vi "startdelayLUT_coMD.vi"() -> ()   [LabVIEW 2012]
doc: "SciScan 1.2 160622"
uses:
  <vilib>/Utility/VariantDataType/Type.ctl
  GFG/GFGbooleanGet.vi
  GFG/GFGfpRefGet.vi
  GFG/GFGstringGet.vi
  GFG/GFG library.lvlib
  <vilib>/Utility/VariantDataType/VariantType.lvlib
panel:
  out "error out 2":errorcluster
  out "error out":errorcluster
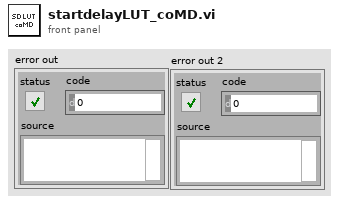
[diagram p1: front panel]
types:
  T1 = cluster{"WaveformChartRef":refnum<vi>, "DigitalRef":refnum<vi>, "ArrayRef":refnum<vi>, "TabControlRef":refnum<vi>, "EnumRef":refnum<vi>, "RingRef":refnum<vi>, "BooleanRef":refnum<vi>, "KnobRef":refnum<vi>, "SlideRef":refnum<vi>, "PathRef":refnum<vi>, "StringRef":refnum<vi>, "ComboBox":refnum<vi>, "WaveformGraphRef":refnum<vi>}
  T2 = enum16{"open", "replace", "create", "open or create", "replace or create", "replace or create with confirmation"}
  T3 = cluster{cluster{"[0]":variant, "[1]":variant, "[2]":variant}[], variant[]}
  T4 = cluster{"params out[0]":variant, "params out[1]":variant, "params out[2]":variant}
  T5 = cluster{"[0]":variant, "[1]":variant, "[2]":variant}[]
  T6 = cluster{"params out[0]":variant, "params out[1]":variant, "params out[2]":variant}[]
  T7 = cluster{cluster{"params out[0]":variant, "params out[1]":variant, "params out[2]":variant}[], variant[]}
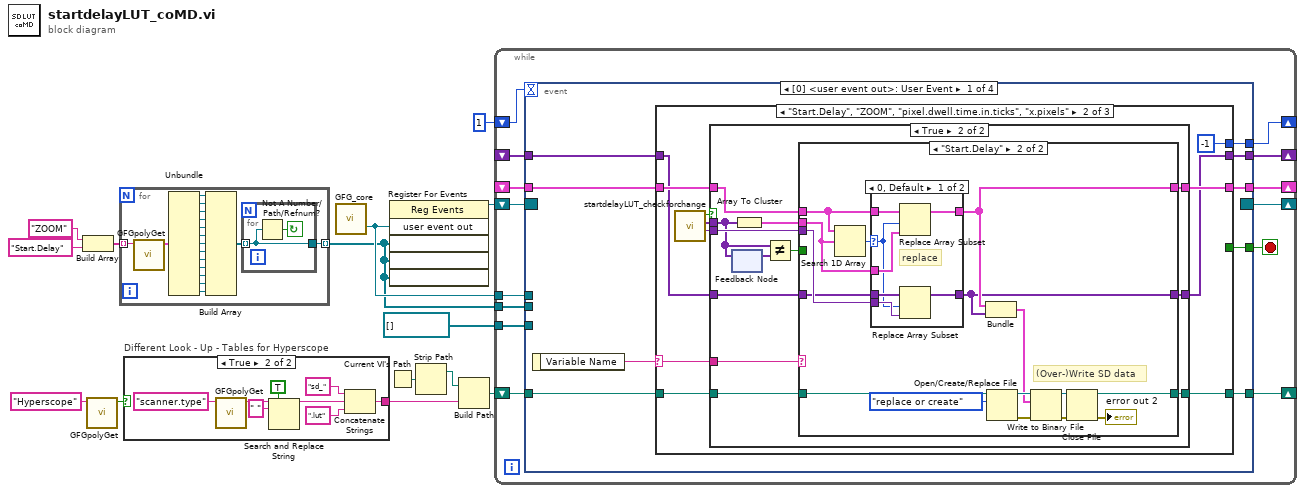
[diagram p0: block diagram]
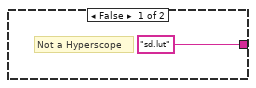
[diagram p2: hidden frame]
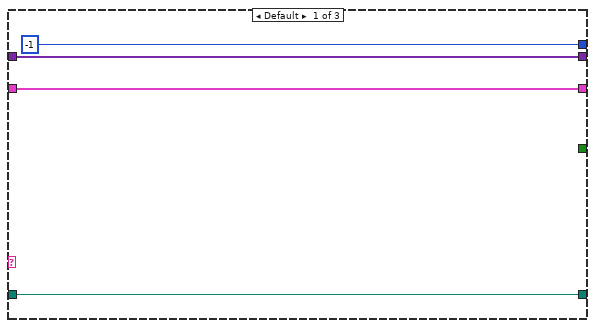
[diagram p3: hidden frame]
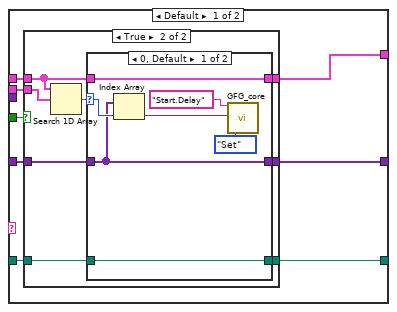
[diagram p5: hidden frame]
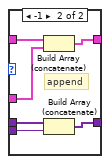
[diagram p8: hidden frame]
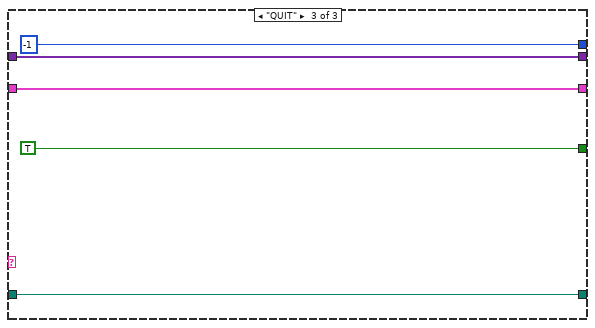
[diagram p9: hidden frame]
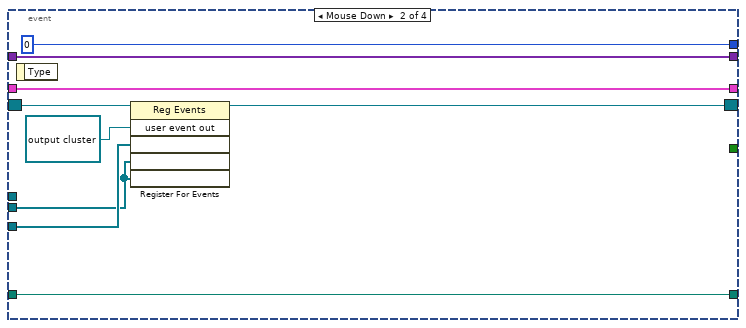
[diagram p10: hidden frame]
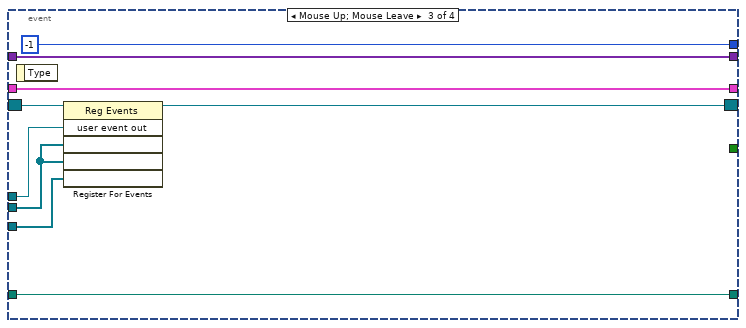
[diagram p11: hidden frame]
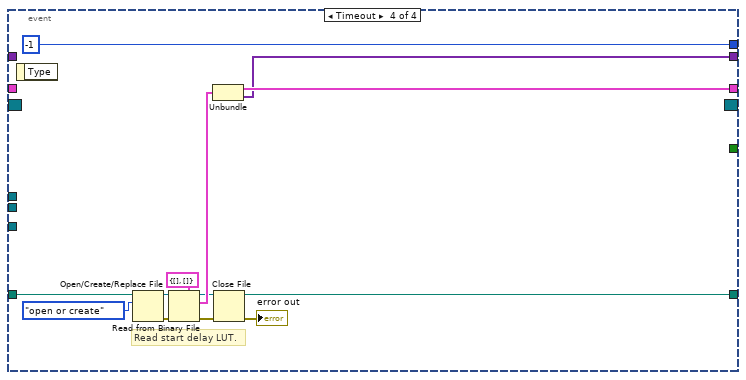
[diagram p12: hidden frame]
diagram:
  n1 = Build Array("ZOOM", "Start.Delay") -> (w10:string[])
  n2 = call-poly "GFGpolyGet.vi"("Variable Name in"="Hyperscope") -> ("Boolean Value OUT"=w3:bool)  [unwired: 9 in, 1 out]
  n3 = for {
    tunnel: w10 -> [w31] mode=indexing
    tunnel: [w15] -> w6 mode=indexing
    n4 = call-poly "GFGpolyGet.vi"("Variable Name in"=w31) -> ("output cluster"=w17:T1)  [unwired: 9 in, 1 out]
    n5 = Unbundle(w17) -> ("WaveformChartRef"=w28:refnum<vi>, "DigitalRef"=w27:refnum<vi>, "ArrayRef"=w26:refnum<vi>, "TabControlRef"=w25:refnum<vi>, "EnumRef"=w24:refnum<vi>, "RingRef"=w23:refnum<vi>, "BooleanRef"=w22:refnum<vi>, "KnobRef"=w21:refnum<vi>, "SlideRef"=w20:refnum<vi>, "PathRef"=w19:refnum<vi>, "StringRef"=w18:refnum<vi>, "ComboBox"=w29:refnum<vi>, "WaveformGraphRef"=w30:refnum<vi>)
    n6 = Build Array(w28, w27, w26, w25, w24, w23, w22, w21, w20, w19, w18, w29, w30) -> (w16:refnum<vi>[])
    n7 = for {
      tunnel: w16 -> [w32] mode=indexing
      tunnel: [w32] -> w15
      stop <- w33 continue-if-true
      n8 = Not A Number/Path/Refnum?(number/path/refnum=w32) -> (NaN/Path/Refnum?=w33:bool)
    }
  }
  n9 = case "Different Look - Up - Tables for Hyperscope" shown="True" w3 {
    tunnel: ["sd.lut" ("name or relative path") w35] -> w1
    frame False {
      # "Not a Hyperscope"
    }
    frame True {
      n10 = call-poly "GFGpolyGet.vi"("Variable Name in"="scanner.type") -> ("String"=w41:string)  [unwired: 9 in, 1 out]
      n11 = Search and Replace String(replace all?=TRUE ("replace all? (F)"), input string=w41, search string=" ") -> (result string=w38:string)  [unwired: 5 in, 3 out]
      n12 = Concatenate Strings("sd_" ("string"), w38, ".lut" ("string")) -> (w35:string)
    }
  }
  n13 = call "GFG_core.vi"() -> ("user event out"=w7:refnum<user-event>)  [unwired: 13 in, 6 out]
  n14 = Current VI's Path() -> (path=w13:path)
  n15 = register-events(w7, w6, w6, w6) -> (reference out=w14:refnum<event-registration>)  [unwired: 2 in, 1 out]
  n16 = Strip Path(path=w13) -> (stripped path=w2:path)  [unwired: 1 out]
  n17 = Build Path(base path=w2, name or relative path=w1) -> (appended path=w12:path)
  n18 = while {
    shift-right: [w52] -> _
    shift-left: _ -> [w53]
    shift-right: [w50] -> _
    shift-left: _ -> [w51]
    shift-right: [w49] -> _
    shift-left: 1 -> [w48]
    tunnel: w6 -> [w47]
    shift-right: [w46] -> _
    shift-left: w14 -> [w56]
    tunnel: w7 -> [w45]
    tunnel: refnum<vi>[] [] ("event source") -> [w44]
    shift-right: [w43] -> _
    shift-left: w12 -> [w55]
    stop <- w54 stop-if-true
    n19 = event shown="[0] <user event out>: User Event" {
      selector: w56 -> [_ w167 w176 _]
      dyn-events: [_ w165 w175 _] -> w46
      timeout: w48 -> [_ _ _ _]
      tunnel: w55 -> [w64 w162 w171 w180]
      tunnel: [w63 _ _ _] -> w54
      tunnel: w53 -> [w62 w160 w168 _]
      tunnel: [w61 w160 w168 w179] -> w52
      tunnel: w51 -> [w60 w159 w170 _]
      tunnel: [w59 w159 w170 w178] -> w50
      tunnel: [w57 0 -1 -1] -> w49
      tunnel: w47 -> [_ w163 w173 _]
      tunnel: w45 -> [_ _ w174 _]
      tunnel: w44 -> [_ w164 w172 _]
      tunnel: [w58 w162 w171 w177] -> w43
      event User Event {
        n20 = event-data() -> ("Variable Name"=w65:string)  [unwired: 1 in]
        n21 = case shown="\"Start.Delay\", \"ZOOM\", \"pixel.dwell.time.in.ticks\", \"x.pixels\"" w65 {
          selector: w65 -> [_ w76 _]
          tunnel: w64 -> [w67 w71 w155]
          tunnel: [_ _ TRUE] -> w63
          tunnel: w62 -> [w68 w80 w156]
          tunnel: [w68 w79 w156] -> w61
          tunnel: w60 -> [w69 w78 w157]
          tunnel: [w69 w77 w157] -> w59
          tunnel: [w67 w70 w155] -> w58
          tunnel: [-1 -1 -1] -> w57
          frame Default {
          }
          frame "Start.Delay", "ZOOM", "pixel.dwell.time.in.ticks", "x.pixels" {
            n22 = call "startdelayLUT_checkforchange.vi"() -> ("start delay out"=w74:variant, "params out"=w73:variant[], "go ahead"=w75:bool)  [unwired: 9 in]
            n23 = case shown="True" w75 {
              tunnel: w71 -> [w81 w94]
              tunnel: w80 -> [w83 w92]
              tunnel: [w83 w91] -> w79
              tunnel: w78 -> [w82 w90]
              tunnel: [w82 w89] -> w77
              tunnel: w76 -> [_ w88]
              tunnel: w74 -> [_ w86]
              tunnel: w73 -> [_ w85]
              tunnel: [w81 w84] -> w70
              frame False {
              }
              frame True {
                n24 = feedback #1() -> (w93:variant[])  [unwired: 1 in]
                n25 = feedback-in #1(w85) -> ()
                n26 = Array To Cluster(array=w85) -> (cluster=w95:T4)
                n27 = Not Equal?(x=w85, y=w93) -> (x != y?=w87:bool)
                n28 = case shown="\"Start.Delay\"" w88 {
                  tunnel: w95 -> [w103 w137]
                  tunnel: w92 -> [w101 w140]
                  tunnel: w86 -> [_ w139]
                  tunnel: [w100 w136] -> w91
                  tunnel: w90 -> [w102 w138]
                  tunnel: w94 -> [w97 w134]
                  tunnel: [w99 w135] -> w89
                  tunnel: w87 -> [w98 _]
                  tunnel: [w96 w133] -> w84
                  frame Default {
                    n29 = case shown="True" w98 {
                      tunnel: w103 -> [_ w113]
                      tunnel: w102 -> [w105 w112]
                      tunnel: w101 -> [w106 w111]
                      tunnel: [w106 w110] -> w100
                      tunnel: [w105 w109] -> w99
                      tunnel: w97 -> [w104 w108]
                      tunnel: [w104 w107] -> w96
                      frame False {
                      }
                      frame True {
                        n30 = Search 1D Array(1D array=w111, element=w113) -> (index of element=w114:i32)  [unwired: 1 in]
                        n31 = case shown="0, Default" w114 {
                          selector: w114 -> [w120 _]
                          tunnel: w111 -> [w121 w124]
                          tunnel: [w121 w124] -> w110
                          tunnel: w112 -> [w119 w123]
                          tunnel: [w119 w123] -> w109
                          tunnel: w108 -> [w115 w122]
                          tunnel: [w115 w122] -> w107
                          frame 0, Default {
                            n32 = Index Array(array=w119, index=w120) -> (element=w116:variant)
                            n33 = call "GFG_core.vi"("Variable Name in"="Start.Delay", "Variant in"=w116, "Action"=enum16{"Init", "Set", "Get", "Clear"}."Set") -> ()  [unwired: 10 in, 7 out]
                          }
                          frame -1 {
                          }
                        }
                      }
                    }
                  }
                  frame "Start.Delay" {
                    # "(Over-)Write SD data"
                    n34 = Search 1D Array(1D array=w140, element=w137) -> (index of element=w132:i32)  [unwired: 1 in]
                    n35 = case shown="0, Default" w132 {
                      selector: w132 -> [w142 _]
                      tunnel: w140 -> [w147 w153]
                      tunnel: w137 -> [w146 w152]
                      tunnel: [w145 w151] -> w136
                      tunnel: w138 -> [w144 w150]
                      tunnel: w139 -> [w143 w148]
                      tunnel: [w141 w149] -> w135
                      frame 0, Default {
                        # "replace"
                        n36 = Replace Array Subset(array=w147, new element=w146, index=w142) -> (w145:T5)
                        n37 = Replace Array Subset(array=w144, new element=w143, index=w142) -> (w141:variant[])
                      }
                      frame -1 {
                        # "append"
                        n38 = Build Array (concatenate)(w153, w152) -> (w151:T6)
                        n39 = Build Array (concatenate)(w150, w148) -> (w149:variant[])
                      }
                    }
                    n40 = Bundle(w136, w135) -> (w126:T7)  [unwired: 1 in]
                    n41 = Open/Create/Replace File(file path (use dialog)=w134, operation (0:open)=T2."replace or create") -> (refnum out=w131:refnum<file>, error out=w128:errorcluster)  [unwired: 4 in, 1 out]
                    n42 = Write to Binary File(file (use dialog)=w131, data=w126, error in=w128) -> (refnum out=w130:refnum<file>, error out=w129:errorcluster)  [unwired: 3 in, 1 out]
                    n43 = Close File(refnum=w130, error in=w129) -> (path=w133:path, error out=→"error out 2":errorcluster)
                  }
                }
              }
            }
          }
          frame "QUIT" {
          }
        }
      }
      event Mouse Down {
        n44 = event-data() -> ()  [unwired: 1 in, 1 out]
        n45 = register-events(reference=w167, refnum<user-event> refnum ("user event out"), w164, w163, w163) -> (reference out=w165:refnum<event-registration>)  [unwired: 1 in, 1 out]
      }
      event Mouse Up; Mouse Leave {
        n46 = event-data() -> ()  [unwired: 1 in, 1 out]
        n47 = register-events(reference=w176, w174, w173, w173, w172) -> (reference out=w175:refnum<event-registration>)  [unwired: 1 in, 1 out]
      }
      event Timeout {
        # "Read start delay LUT."
        n48 = event-data() -> ()  [unwired: 1 in, 1 out]
        n49 = Open/Create/Replace File(file path (use dialog)=w180, operation (0:open)=T2."open or create") -> (refnum out=w187:refnum<file>, error out=w183:errorcluster)  [unwired: 4 in, 1 out]
        n50 = Read from Binary File(5:T3 {[], []} ("output cluster"), 8:w183, 11:w187) -> (0:w184:errorcluster, 2:w188:T3, 3:w185:refnum<file>)  [unwired: 3 in, 1 out]
        n51 = Unbundle(w188) -> (w179:T5, w178:variant[])
        n52 = Close File(refnum=w185, error in=w184) -> (path=w177:path, error out=→"error out":errorcluster)
      }
    }
  }
